vi "Configure CALC2 Input Path.vi"(8 "error in (no error)":errorcluster, 10 "Limit Test Source (0: SENSE)":u16(ring) items=["Measurements (SENSE)", "Math Calculations (CALC1)"], 11 "VISA resource name":refnum<visa-resource-name>) -> (0 "error out":errorcluster, 3 "VISA resource name out":refnum<visa-resource-name>)   [LabVIEW 2020, in "Keithley 6517.lvlib"]
doc: "Configures Limit Testing input path.\n\n<B>Note:</B>\nThis VI is ONLY compatible with <B>model 6514</B>. Running this VI with any other model will result in an error."
uses:
  <instrlib>/Keithley 6517/Keithley 6517.lvlib
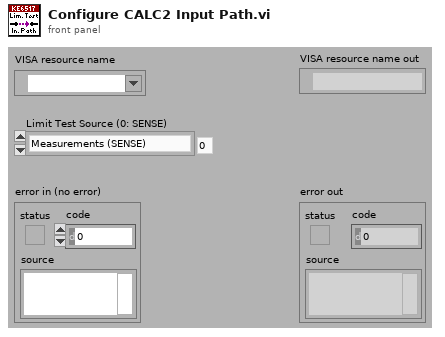
[diagram p1: front panel]
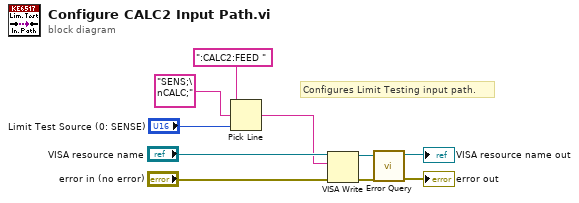
[diagram p0: block diagram]
diagram:
  # "Configures Limit Testing input path."
  n1 = Pick Line(string ("")=":CALC2:FEED ", multi-line string="SENS;\nCALC;", line index="Limit Test Source (0: SENSE)") -> (output string=w5:string)
  n2 = VISA Write(VISA resource name="VISA resource name", write buffer=w5, error in (no error)="error in (no error)") -> (VISA resource name out=w1:refnum<visa-resource-name>, error out=w4:errorcluster)  [unwired: 1 out]
  n3 = call <instrlib>:"Error Query.vi"("error in (no error)"=w4, "VISA resource name"=w1) -> ("error out"=→"error out":errorcluster, "VISA resource name out"=→"VISA resource name out":refnum<visa-resource-name>)  [unwired: 6 in, 2 out]
